vi "LVClass_ClosedLoopSecurity_GetData.vi"(0 "ClosedLoopSecurity in":refnum<class "ClosedLoopSecurity.lvclass">, 11 "error in (no error)":errorcluster) -> (4 "ClosedLoopSecurity out":refnum<class "ClosedLoopSecurity.lvclass">, 6 "ClosedLoopSecurityParams":T1, 15 "error out":errorcluster)   [LabVIEW 2020, in "ClosedLoopSecurity.lvclass"]
doc: "get tolerances\n\n<B>security_paramsIn</B> : Pointer to Closed Loop security params object.\n<B>security_paramsOut</B> : Pointer to Closed Loop security params object.\n<B>max_saturated_act_count</B> : Maximum tolerated count of saturated actuators\n<B>max_camera_fill_pct</B> : Maximum tolerated saturation percentage on camera signal\n<B>max_pupil_size_variation</B> : Maximum tolerated variation of the pupil size, relatively to the command\n matrix pupil size\n<B>max_dwf_pv</B> : Maximum tolerated loop smoothing gain"
uses:
  ClosedLoopSecurity.lvclass
  ClosedLoopSecurityParameters.ctl
  ClosedLoopSecurity.lvclass/ClosedLoopSecurity.ctl
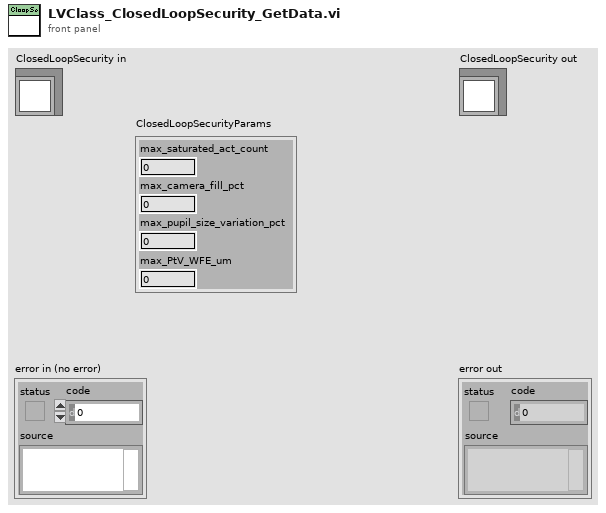
[diagram p1: front panel]
types:
  T1 = typedef "ClosedLoopSecurityParameters.ctl" = cluster{"max_saturated_act_count":i32, "max_camera_fill_pct":i32, "max_pupil_size_variation_pct":i32, "max_PtV_WFE_um":sgl}
  T2 = typedef "ClassID.ctl" = i64
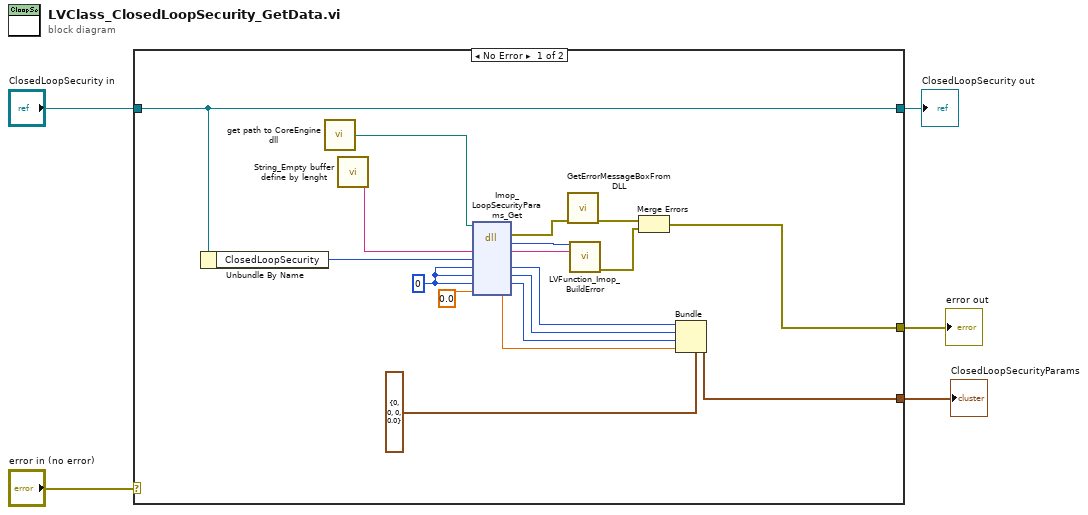
[diagram p0: block diagram]
diagram:
  n1 = case shown="No Error" "error in (no error)" {
    selector: "error in (no error)" -> [_ w25]
    tunnel: [w16 w25] -> w4
    tunnel: [w14 w24] -> w2
    tunnel: "ClosedLoopSecurity in" -> [w14 w24]
    tunnel: [w9 _] -> w1
    frame No Error {
      w7 = 0 ("High_amplitude")
      n2 = Unbundle By Name(w14) -> ("ClosedLoopSecurity"=w15:T2)
      n3 = call "get path to CoreEngine dll.vi"() -> ("path to wavekit library"=w17:path)  [unwired: 14 in, 1 out]
      n4 = call "String_Empty buffer define by lenght.vi"() -> ("Empty buffer"=w23:string)  [unwired: 1 in]
      n5 = dll-call lib="D:/soft/HASO_v3/SVN_trunk/ImOpCoreEngine4_LV2011/DLLs/c_interface_vc100.dll" fn="Imop_LoopSecurityParams_Get"(path in=w17, "message"=w23, "security_params"=w15, "max_saturated_act_count"=w7, "max_camera_fill_pct"=w7, "max_pupil_size_variation"=w7, "max_loop_gain"=sgl 0.0 ("low_gain_factor")) -> (error out=w20:errorcluster, "return type"=w21:i32, "message"=w22:string, "max_saturated_act_count"=w13:i32, "max_camera_fill_pct"=w12:i32, "max_pupil_size_variation"=w11:i32, "max_loop_gain"=w10:sgl)  [unwired: 3 in, 1 out]
      n6 = call "GetErrorMessageBoxFromDLL.vi"("error IN"=w20) -> ("error OUT"=w19:errorcluster)  [unwired: 10 in]
      n7 = call "LVFunction_Imop_BuildError.vi"("code"=w21, "String to Prepend to source (\"\")"=w22) -> ("error out"=w18:errorcluster)  [unwired: 13 in]
      n8 = Merge Errors(w19, w18) -> (w16:errorcluster)
      n9 = Bundle(cluster=T1 {"max_saturated_act_count"=0, "max_camera_fill_pct"=0, "max_pupil_size_variation_pct"=0, "max_PtV_WFE_um"=0.0} ("ClosedLoopSecurityParams"), "max_saturated_act_count"=w13, "max_camera_fill_pct"=w12, "max_pupil_size_variation_pct"=w11, "max_PtV_WFE_um"=w10) -> (w9:T1)
    }
    frame Error {
    }
  }
  "error out" <- w4
  "ClosedLoopSecurity out" <- w2
  "ClosedLoopSecurityParams" <- w1
